vi "OPEN & CONFIG ARMS.vi"(0 "LEFT or RIGHT":string="LEFT", 1 "CLIMBER COAST":T2=enum."Override to Brake", 5 "CLIMBER CAN ID":u8=9, 7 "LOCK PWM channel":T1=enum."PWM 2", 9 "ARM CAN ID":u8=11, 11 "error in (no error)":errorcluster, 12 "Invert climber?":bool, 14 "Invert arm actuator?":bool) -> (15 "error out":errorcluster)   [LabVIEW 2020]
uses:
  <vilib>/Rock Robotics/WPI/ThirdParty/Phoenix-LabVIEW/Motor Controller/Controls/CTRE_Phoenix_MotorControl_TalonFXMotorControllerConfigurables.ctl
  <vilib>/Rock Robotics/WPI/ThirdParty/Phoenix-LabVIEW/Motor Controller/Controls/CTRE_Phoenix_MotorControl_BaseConfigurables.ctl
  <vilib>/Rock Robotics/WPI/ThirdParty/Phoenix-LabVIEW/Motor Controller/Controls/CTRE_Phoenix_MotorControl_VelocityMeasurementPeriod.ctl
  <vilib>/Rock Robotics/WPI/ThirdParty/Phoenix-LabVIEW/Motor Controller/Controls/CTRE_Phoenix_MotorControl_SlotStructure.ctl
  <vilib>/Rock Robotics/WPI/ThirdParty/Phoenix-LabVIEW/Motor Controller/Controls/CTRE_Phoenix_MotorControl_FilterStruct.ctl
  <vilib>/Rock Robotics/WPI/ThirdParty/Phoenix-LabVIEW/Motor Controller/Controls/CTRE_Phoenix_MotorControl_RemoteSourceType.ctl
  <vilib>/Rock Robotics/WPI/ThirdParty/Phoenix-LabVIEW/Controls/CTRE_Phoenix_CustomParamConfiguration.ctl
  <vilib>/Rock Robotics/WPI/ThirdParty/Phoenix-LabVIEW/Motor Controller/Controls/CTRE_Phoenix_MotorControl_FeedbackDevice_TalonFX.ctl
  <vilib>/Rock Robotics/WPI/ThirdParty/Phoenix-LabVIEW/Motor Controller/Controls/CTRE_Phoenix_MotorControl_LimitSwitchNormal.ctl
  <vilib>/Rock Robotics/WPI/ThirdParty/Phoenix-LabVIEW/Motor Controller/Controls/CTRE_Phoenix_MotorControl_LimitSwitchSource_Local.ctl
  <vilib>/Rock Robotics/WPI/ThirdParty/Phoenix-LabVIEW/Motor Controller/Controls/CTRE_Phoenix_MotorControl_SupplyCurrentLimitConfiguration.ctl
  <vilib>/Rock Robotics/WPI/ThirdParty/Phoenix-LabVIEW/Motor Controller/Controls/CTRE_Phoenix_MotorControl_StatorCurrentLimitConfiguration.ctl
  <vilib>/Rock Robotics/WPI/ThirdParty/Phoenix-LabVIEW/Motor Controller/Controls/CTRE_Phoenix_MotorControl_MotorCommutation_TalonFX.ctl
  <vilib>/Rock Robotics/WPI/ThirdParty/Phoenix-LabVIEW/CANCoder/Controls/CTRE_Phoenix_CANcoder_AbsoluteSensorRange.ctl
  <vilib>/Rock Robotics/WPI/ThirdParty/Phoenix-LabVIEW/CANCoder/Controls/CTRE_Phoenix_CANcoder_SensorInitializationStrategy.ctl
  <vilib>/Rock Robotics/WPI/ThirdParty/Phoenix-LabVIEW/Motor Controller/Controls/CTRE_Phoenix_MotorControl_NeutralMode.ctl
  <vilib>/Rock Robotics/SystemInterfaces/DIO/FPGA_DIOPWMChannel.ctl
  <vilib>/Rock Robotics/WPI/SafetyOutput/WPI_SafetyOutputConfigMenu.ctl
  Robot Global Data.vi
  <vilib>/Rock Robotics/Network Tables/NT Write Number.vi
  <vilib>/Rock Robotics/Network Tables/NT Write Boolean.vi
panel:
  in  "FALCON Climbing config":T3={"Base Configurables"={"openLoopRamp"=0.25, "closedLoopRamp"=0.125, "peakOutputForward"=1.0, "peakOutputReverse"=-1.0, "nominalOutputForward"=0.0, "nominalOutputReverse"=0.0, "neutralDeadband"=0.04, "voltageCompSaturation"=0.0, "voltageMeasurementFilter"=32, "velocityMeasurementPeriod"=100, "velocityMeasurementWindow"=64, "forwardSoftLimitThreshold"=441205, "reverseSoftLimitThreshold"=0, "forwardSoftLimitEnable"=TRUE, "reverseSoftLimitEnable"=TRUE, "slot0"={"P"=0.0, "I"=0.0, "D"=0.0, "F"=0.0, "integralZone"=0.0, "allowableClosedLoopError"=0, "maxIntegralAccumulator"=0.0, "closedLoopPeakOutput"=1.0, "closedLoopPeriod"=1}, "slot1"={"P"=0.0, "I"=0.0, "D"=0.0, "F"=0.0, "integralZone"=0.0, "allowableClosedLoopError"=0, "maxIntegralAccumulator"=0.0, "closedLoopPeakOutput"=1.0, "closedLoopPeriod"=1}, "slot2"={"P"=0.0, "I"=0.0, "D"=0.0, "F"=0.0, "integralZone"=0.0, "allowableClosedLoopError"=0, "maxIntegralAccumulator"=0.0, "closedLoopPeakOutput"=1.0, "closedLoopPeriod"=1}, "slot3"={"P"=0.0, "I"=0.0, "D"=0.0, "F"=0.0, "integralZone"=0.0, "allowableClosedLoopError"=0, "maxIntegralAccumulator"=0.0, "closedLoopPeakOutput"=1.0, "closedLoopPeriod"=1}, "auxPIDPolarity"=FALSE, "remoteFilter0"={"remoteSensorDeviceID"=0, "remoteSensorSource"=enum."Off"}, "remoteFilter1"={"remoteSensorDeviceID"=0, "remoteSensorSource"=enum."Off"}, "motionCruiseVelocity"=0, "motionAcceleration"=0, "motionProfileTrajectoryPeriod"=0, "feedbackNotContinuous"=FALSE, "remoteSensorClosedLoopDisableNeutralOnLOS"=FALSE, "clearPositionOnLimitF"=FALSE, "clearPositionOnLimitR"=FALSE, "clearPositionOnQuadIdx"=FALSE, "limitSwitchDisableNeutralOnLOS"=FALSE, "softLimitDisableNeutralOnLOS"=FALSE, "pulseWidthPeriod_EdgesPerRot"=1, "pulseWidthPeriod_FilterWindowSz"=1, "customParam"={"customParam0"=0, "customParam1"=0}, "trajectoryInterpolationEnable"=TRUE}, "primaryPID"={"selectedFeedbackCoefficient"=1.0, "selectedFeedbackSensor"=1}, "auxiliaryPID"={"selectedFeedbackCoefficient"=1.0, "selectedFeedbackSensor"=1}, "forwardLimitSwitchNormal"=enum."Normally Open", "reverseLimitSwitchNormal"=enum."Normally Open", "forwardLimitSwitchDeviceID"=0, "reverseLimitSwitchDeviceID"=0, "forwardLimitSwitchSource"=enum."Feedback Connector", "reverseLimitSwitchSource"=enum."Feedback Connector", "sum0Term"=1, "sum1Term"=1, "diff0Term"=1, "diff1Term"=1, "Supply Current Limit Configuration"={"Enable?"=FALSE, "Current Limit"=0.0, "Threshold Current"=0.0, "Threshold Time"=0.0}, "Stator Current Limit Configuration"={"Enable?"=FALSE, "Current Limit"=0.0, "Threshold Current"=0.0, "Threshold Time"=0.0}, "Motor Commutation"=enum."Trapezoidal", "Absolute Sensor Range"=enum."Unsigned [0 to 360)", "Integrated Sensor Offset (Degrees)"=0.0, "Sensor Initialization Strategy"=enum."Boot To Zero"} {"diff1Term" items=["Integrated Sensor"=1, "Sensor Sum (S0 + S1)"=9, "Sensor Difference (D0 - D1)"=10, "Remote Source 0"=11, "Remote Source 1"=12, "None"=14, "Software Emulated"=15]; "diff0Term" items=["Integrated Sensor"=1, "Sensor Sum (S0 + S1)"=9, "Sensor Difference (D0 - D1)"=10, "Remote Source 0"=11, "Remote Source 1"=12, "None"=14, "Software Emulated"=15]; "sum1Term" items=["Integrated Sensor"=1, "Sensor Sum (S0 + S1)"=9, "Sensor Difference (D0 - D1)"=10, "Remote Source 0"=11, "Remote Source 1"=12, "None"=14, "Software Emulated"=15]; "sum0Term" items=["Integrated Sensor"=1, "Sensor Sum (S0 + S1)"=9, "Sensor Difference (D0 - D1)"=10, "Remote Source 0"=11, "Remote Source 1"=12, "None"=14, "Software Emulated"=15]; "auxiliaryPID"."selectedFeedbackSensor" items=["Integrated Sensor"=1, "Sensor Sum (S0 + S1)"=9, "Sensor Difference (D0 - D1)"=10, "Remote Source 0"=11, "Remote Source 1"=12, "None"=14, "Software Emulated"=15]; "primaryPID"."selectedFeedbackSensor" items=["Integrated Sensor"=1, "Sensor Sum (S0 + S1)"=9, "Sensor Difference (D0 - D1)"=10, "Remote Source 0"=11, "Remote Source 1"=12, "None"=14, "Software Emulated"=15]; "Base Configurables"."velocityMeasurementPeriod" items=["Period_1ms"=1, "Period_2ms"=2, "Period_5ms"=5, "Period_10ms"=10, "Period_20ms"=20, "Period_25ms"=25, "Period_50ms"=50, "Period_100ms"=100]}
  # "Climbing soft limit calc:\n23.5\" max travel\n1.25\" diameter sprocket\n36:1 planetary gearbox\n2048 encoder tics/rev for a Falcon 500\n\n23.5 in * rev/(pi*1.25\") * 36 motor rev/rev * 2048 tics/motor rev = 441205 tics"
  # "Sum and Diff terms are ways to select more than one sensor as a feedback device. \n Sum 0 is the first feedback device to be used for the Sum term.\n Sum 1 is the feedback device to be added to Sum 0 for the Sum term.\n Diff 0 and Diff 1 work in a similar manner."
  # "These are only applicable\nif using a remote limit switch.\n\nLocal limit switches/no limit\nswitches do not use this."
  # "Current is below Current Limit AND\n\n(Requested output is weaker** than applied motor\noutput OR is in the opposite direction).\n/\nMotor output is set to requested output."
  # "Current is above Threshold Current for Threshold Time\n/\nReduce motor output (towards neutral)."
  # "Current is below Current Limit.\n/\nRamp motor output towards requested output."
  # "Current is above Current Limit.\n/\nReduce motor output (towards neutral)."
  # "*If the configured Peak Threshold is less than the Continuous Threshold, the applied Peak Threshold is set equal to the Configured Continuous Threshold in firmware.\n** Both requested output and applied motor output are in the same direction, and requested output is closer to neutral."
  # "False: Primary Output = PID[0] + PID[1]  ---  Auxiliary Output = PID[0] - PID[1]\nTrue:  Primary Output = PID[0] - PID[1] --- Auxiliary Output = PID[0] + PID[1]"
  # "Enable the motion profile executor to perform linear interpolation between profile points.  Defaults to True."
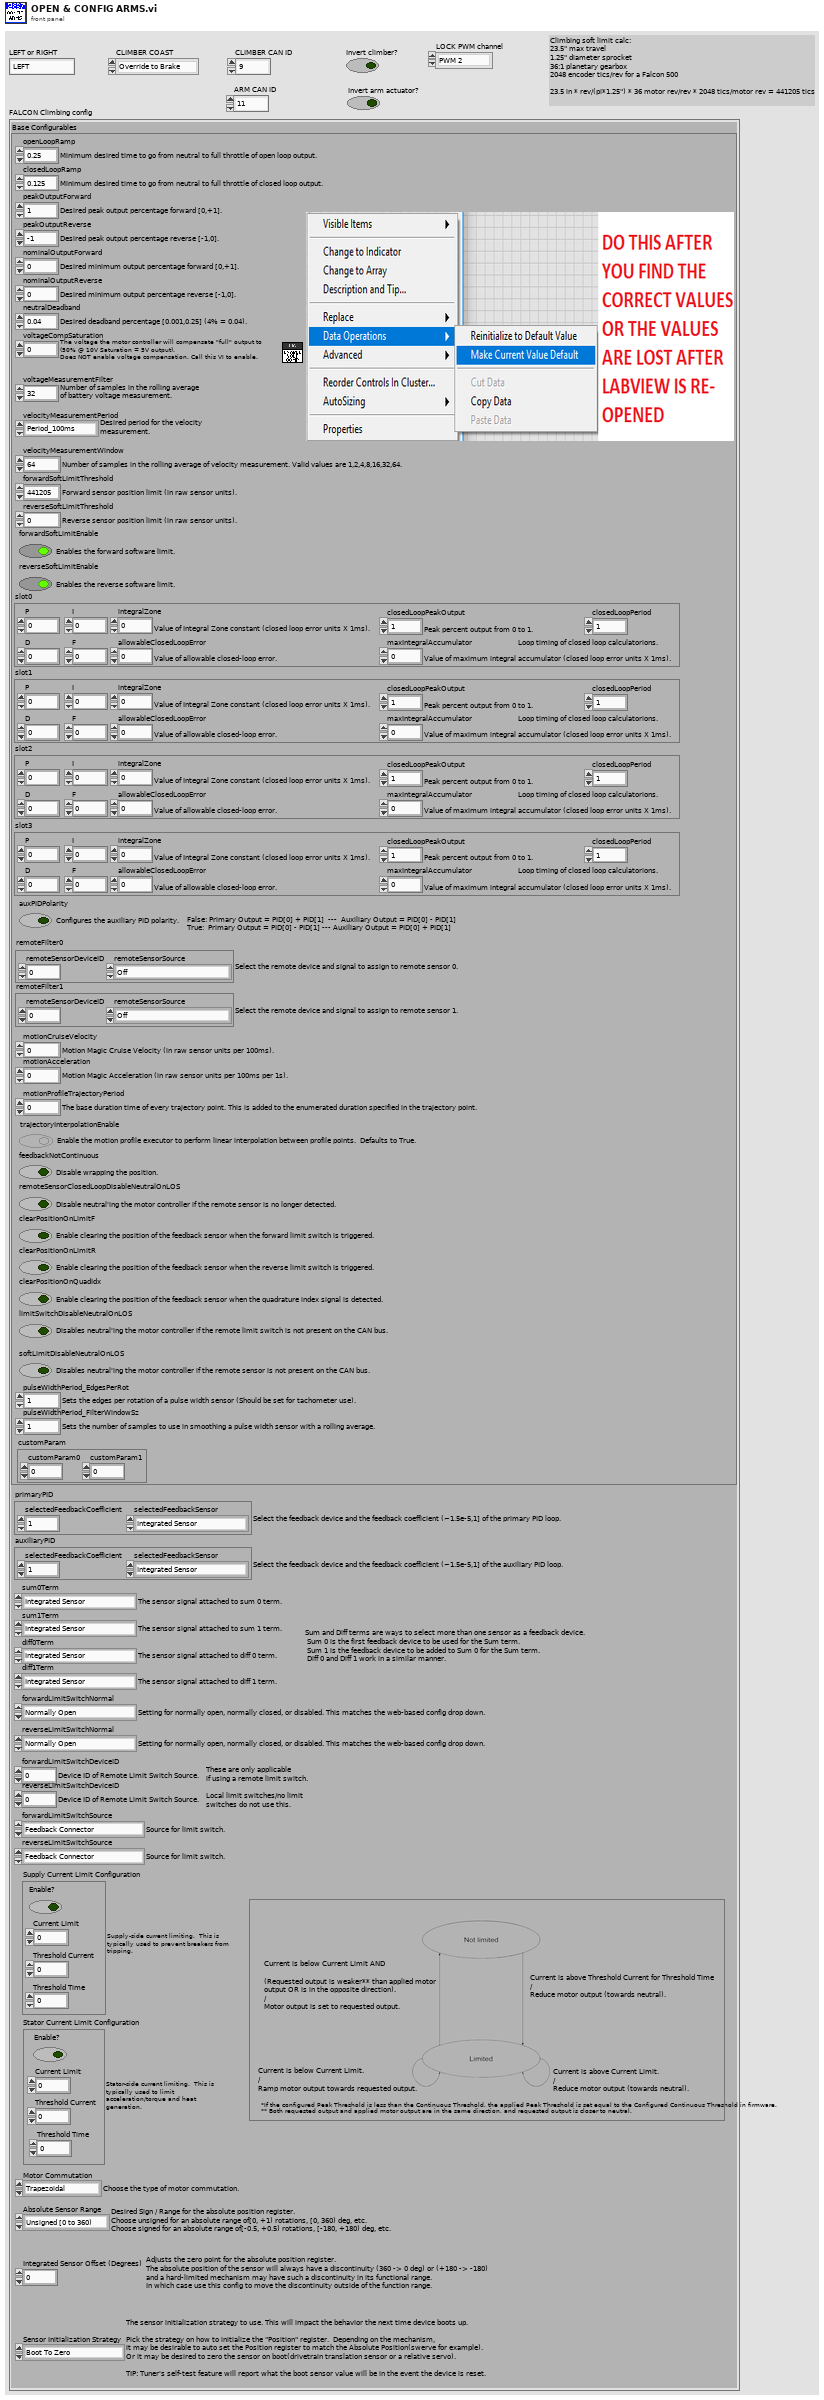
[diagram p1: front panel]
types:
  T1 = typedef "FPGA_DIOPWMChannel.ctl" = enum8{"PWM 0", "PWM 1", "PWM 2", "PWM 3", "PWM 4", "PWM 5", "PWM 6", "PWM 7", "PWM 8", "PWM 9", "PWM MXP 0", "PWM MXP 1", "PWM MXP 2", "PWM MXP 3", "PWM MXP 4", "PWM MXP 5", "PWM MXP 6", "PWM MXP 7", "PWM MXP 8", "PWM MXP 9", "Invalid"}
  T2 = typedef "CTRE_Phoenix_MotorControl_NeutralMode.ctl" = enum8{"EEPROMSetting", "Override to Coast", "Override to Brake"}
  T3 = typedef "CTRE_Phoenix_MotorControl_TalonFXMotorControllerConfigurables.ctl" = cluster{"Base Configurables":T4, "primaryPID":cluster{"selectedFeedbackCoefficient":dbl, "selectedFeedbackSensor":T10}, "auxiliaryPID":cluster{"selectedFeedbackCoefficient":dbl, "selectedFeedbackSensor":T10}, "forwardLimitSwitchNormal":T11, "reverseLimitSwitchNormal":T11, "forwardLimitSwitchDeviceID":i32, "reverseLimitSwitchDeviceID":i32, "forwardLimitSwitchSource":T12, "reverseLimitSwitchSource":T12, "sum0Term":T10, "sum1Term":T10, "diff0Term":T10, "diff1Term":T10, "Supply Current Limit Configuration":T13, "Stator Current Limit Configuration":T14, "Motor Commutation":T15, "Absolute Sensor Range":T16, "Integrated Sensor Offset (Degrees)":dbl, "Sensor Initialization Strategy":T17}
  T4 = typedef "CTRE_Phoenix_MotorControl_BaseConfigurables.ctl" = cluster{"openLoopRamp":dbl, "closedLoopRamp":dbl, "peakOutputForward":dbl, "peakOutputReverse":dbl, "nominalOutputForward":dbl, "nominalOutputReverse":dbl, "neutralDeadband":dbl, "voltageCompSaturation":dbl, "voltageMeasurementFilter":i32, "velocityMeasurementPeriod":T5, "velocityMeasurementWindow":i32, "forwardSoftLimitThreshold":i32, "reverseSoftLimitThreshold":i32, "forwardSoftLimitEnable":bool, "reverseSoftLimitEnable":bool, "slot0":T6, "slot1":T6, "slot2":T6, "slot3":T6, "auxPIDPolarity":bool, "remoteFilter0":T7, "remoteFilter1":T7, "motionCruiseVelocity":i32, "motionAcceleration":i32, "motionProfileTrajectoryPeriod":i32, "feedbackNotContinuous":bool, "remoteSensorClosedLoopDisableNeutralOnLOS":bool, "clearPositionOnLimitF":bool, "clearPositionOnLimitR":bool, "clearPositionOnQuadIdx":bool, "limitSwitchDisableNeutralOnLOS":bool, "softLimitDisableNeutralOnLOS":bool, "pulseWidthPeriod_EdgesPerRot":i32, "pulseWidthPeriod_FilterWindowSz":i32, "customParam":T9, "trajectoryInterpolationEnable":bool}
  T5 = typedef "CTRE_Phoenix_MotorControl_VelocityMeasurementPeriod.ctl" = u16
  T6 = typedef "CTRE_Phoenix_MotorControl_SlotStructure.ctl" = cluster{"P":dbl, "I":dbl, "D":dbl, "F":dbl, "integralZone":dbl, "allowableClosedLoopError":i32, "maxIntegralAccumulator":dbl, "closedLoopPeakOutput":dbl, "closedLoopPeriod":i32}
  T7 = typedef "CTRE_Phoenix_MotorControl_FilterStruct.ctl" = cluster{"remoteSensorDeviceID":u8, "remoteSensorSource":T8}
  T8 = typedef "CTRE_Phoenix_MotorControl_RemoteSourceType.ctl" = enum16{"Off", "Talon SRX Selected Sensor", "Pigeon IMU Yaw", "Pigeon IMU Pitch", "Pigeon IMU Roll", "CANifier Quadrature", "CANifier PWM Input 0", "CANifier PWM Input 1", "CANifier PWM Input 2", "CANifier PWM Input 3", "Gadgeteer Pigeon Yaw", "Gadgeteer Pigeon Pitch", "Gadgeteer Pigeon Roll", "CANCoder"}
  T9 = typedef "CTRE_Phoenix_CustomParamConfiguration.ctl" = cluster{"customParam0":i32, "customParam1":i32}
  T10 = typedef "CTRE_Phoenix_MotorControl_FeedbackDevice_TalonFX.ctl" = i8
  T11 = typedef "CTRE_Phoenix_MotorControl_LimitSwitchNormal.ctl" = enum16{"Normally Open", "Normally Closed", "Disabled"}
  T12 = typedef "CTRE_Phoenix_MotorControl_LimitSwitchSource_Local.ctl" = enum16{"Feedback Connector", "Remote Talon SRX", "Remote CANifier", "Deactivated"}
  T13 = typedef "CTRE_Phoenix_MotorControl_SupplyCurrentLimitConfiguration.ctl" = cluster{"Enable?":bool, "Current Limit":dbl, "Threshold Current":dbl, "Threshold Time":dbl}
  T14 = typedef "CTRE_Phoenix_MotorControl_StatorCurrentLimitConfiguration.ctl" = cluster{"Enable?":bool, "Current Limit":dbl, "Threshold Current":dbl, "Threshold Time":dbl}
  T15 = typedef "CTRE_Phoenix_MotorControl_MotorCommutation_TalonFX.ctl" = enum16{"Trapezoidal"}
  T16 = typedef "CTRE_Phoenix_CANcoder_AbsoluteSensorRange.ctl" = enum16{"Unsigned [0 to 360)", "Signed [-180 to +180)"}
  T17 = typedef "CTRE_Phoenix_CANcoder_SensorInitializationStrategy.ctl" = enum16{"Boot To Zero", "Boot To Absolute Position"}
  T18 = typedef "WPI_SafetyOutputConfigMenu.ctl" = enum16{"Enable", "Disable"}
  T19 = typedef "WPI_MotorControlDeviceRef.ctl" = cluster{"DeviceStatus":errorcluster, "Type":T20, "PWM":cluster{"PWM Channel":T1, "DeadBand":T21}, "CAN":cluster{"Device Number":u8, "SetOutput VI Ref":variant, "GetOutput VI Ref":variant, "Enable VI Ref":variant, "Disable VI Ref":variant, "Data":variant}, "Invert":bool, "DIO PWM":cluster{"PWM \"Enable\" Channel":T1, "DIOChannel":T22, "PWM Rate":dbl}}
  T20 = typedef "WPI_MotorControlType.ctl" = enum16{"PWM", "CAN", "DIO PWM"}
  T21 = typedef "WPI_PWMDeadband.ctl" = cluster{"Name":string, "maxPositivePwm":i32, "minPositivePwm":i32, "centerPwm":i32, "maxNegativePwm":i32, "minNegativePwm":i32, "angularRange":u16}
  T22 = typedef "FPGA_DIOChannel.ctl" = enum8{"DIO 0", "DIO 1", "DIO 2", "DIO 3", "DIO 4", "DIO 5", "DIO 6", "DIO 7", "DIO 8", "DIO 9", "DIO MXP 0", "DIO MXP 1", "DIO MXP 2", "DIO MXP 3", "DIO MXP 4", "DIO MXP 5", "DIO MXP 6", "DIO MXP 7", "DIO MXP 8", "DIO MXP 9", "DIO MXP 10", "DIO MXP 11", "DIO MXP 12", "DIO MXP 13", "DIO MXP 14", "DIO MXP 15", "SPI Port CS1", "SPI Port CS2", "SPI Port CS3", "SPI Port MISO", "SPI Port MOSI", "Invalid"}
  T23 = cluster{"MIN":dbl, "MAX":dbl, "convert climber inches to tics":dbl}
  T24 = cluster{"RANGE":u16, "UNLOCKED angle":i32, "LOCKED angle":i32}
  T25 = typedef "WPI_ServoDeviceRef.ctl" = cluster{"DeviceStatus":errorcluster, "PWM Channel":T1, "DeadBand":T21}
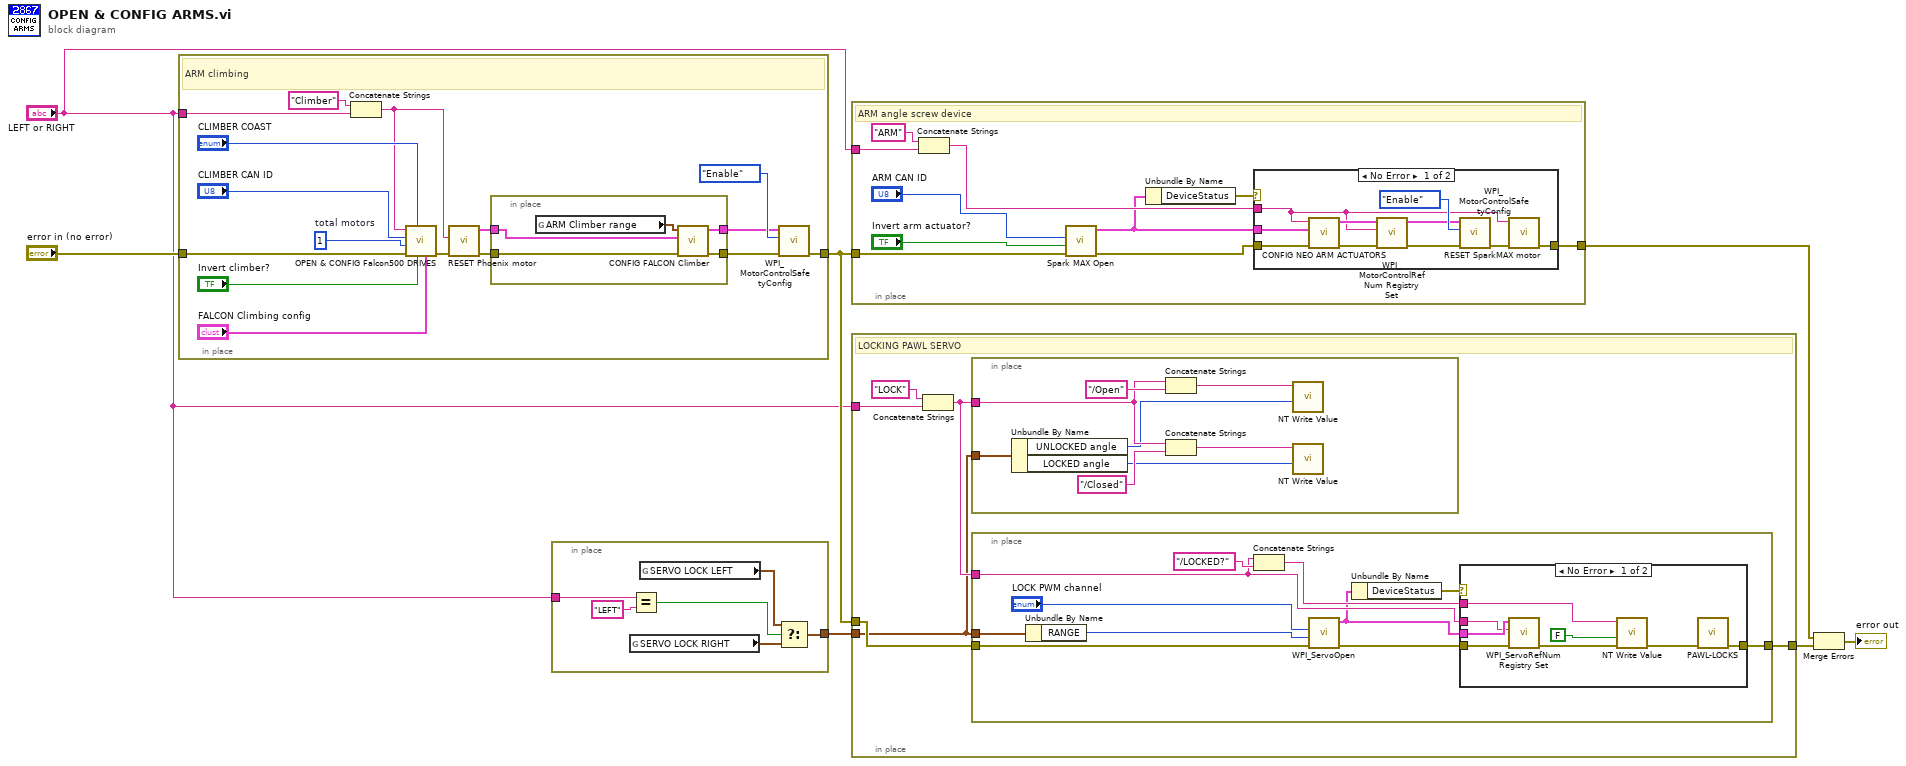
[diagram p0: block diagram]
diagram:
  n1 = in-place {
    in-place-border: "error in (no error)" -> [w14]
    in-place-border: "LEFT or RIGHT" -> [w23]
    in-place-border: [w21] -> w5
    w18 = 1  # total motors
    # "ARM climbing"
    n2 = Concatenate Strings("Climber" ("refnum name"), w23) -> (w12:string)
    n3 = call "OPEN & CONFIG Falcon500 DRIVES.vi"("Talon FX Configurables"="FALCON Climbing config", "INVERT motors?"="Invert climber?", "Motor Control Neutral Mode"="CLIMBER COAST", "error in"=w14, "total motors"=w18, "CAN ID for MASTER DRIVE"="CLIMBER CAN ID", "MASTER DRIVE REF name"=w12) -> ("error out"=w13:errorcluster)  [unwired: 2 in, 2 out]
    n4 = call "RESET Phoenix motor.vi"("error in (no error)"=w13, "Phoenix motor refname"=w12) -> ("error out"=w9:errorcluster, "PhoenixMotorControlDevRef"=w11:T19)  [unwired: 6 in, 2 out]
    n5 = in-place {
      in-place-border: w11 -> [w28]
      in-place-border: [w26] -> w10
      in-place-border: w9 -> [w25]
      in-place-border: [w24] -> w8
      n6 = global read "Robot Global Data.vi" "ARM Climber range"() -> (w27:T23)
      n7 = call "CONFIG FALCON Climber.vi"("error in (no error)"=w25, "PhoenixMotorControlDevRef in"=w28, "ARM Climber range"=w27) -> ("error out"=w24:errorcluster, "PhoenixMotorControlDevRef out"=w26:T19)  [unwired: 7 in]
    }
    n8 = call <vilib>:"WPI_MotorControlSafetyConfig.vi"("error in (no error)"=w8, "mode"=WPI_SafetyOutputConfigMenu."Enable", "MotorControlDevRef"=w10) -> ("error out"=w21:errorcluster)  [unwired: 7 in, 1 out]
  }
  n9 = in-place {
    in-place-border: "LEFT or RIGHT" -> [w33]
    in-place-border: [w29] -> w1
    n10 = global read "Robot Global Data.vi" "SERVO LOCK RIGHT"() -> (w30:T24)
    n11 = Equal?(x=w33, y="LEFT") -> (x = y?=w34:bool)
    n12 = global read "Robot Global Data.vi" "SERVO LOCK LEFT"() -> (w31:T24)
    n13 = Select(t=w31, s=w34, f=w30) -> (s? t:f=w29:T24)
  }
  n14 = in-place "In Place Element Structure" {
    in-place-border: "LEFT or RIGHT" -> [w44]
    in-place-border: [w38] -> w6
    in-place-border: w5 -> [w42]
    # "ARM angle screw device"
    n15 = Concatenate Strings("ARM" ("refnum name"), w44) -> (w37:string)
    n16 = call <vilib>:"Spark MAX Open.vi"("error in (no error)"=w42, "Invert"="Invert arm actuator?", "Device Number"="ARM CAN ID") -> ("error out"=w39:errorcluster, "MotorControlDeviceRef"=w35:T19)  [unwired: 7 in]
    n17 = Unbundle By Name(w35) -> ("DeviceStatus"=w36:errorcluster)
    n18 = case shown="No Error" w36 {
      tunnel: w39 -> [w51 _]
      tunnel: w35 -> [w50 _]
      tunnel: [w46 _] -> w38
      tunnel: w37 -> [w45 _]
      frame No Error {
        n19 = call "CONFIG NEO ARM ACTUATORS.vi"("error in (no error)"=w51, "MotorControlDevRef"=w50, "RefName"=w45) -> ("error out"=w52:errorcluster, "MotorControlDeviceRef out"=w49:T19)  [unwired: 7 in]
        n20 = call <vilib>:"WPI_MotorControlRefNum Registry Set.vi"("error in (no error)"=w52, "refnum name"=w45, "MotorControlDevRef"=w49) -> ("error out"=w48:errorcluster, "MotorControlDevRef"=w53:T19)  [unwired: 7 in]
        n21 = call <vilib>:"WPI_MotorControlSafetyConfig.vi"("error in (no error)"=w48, "mode"=WPI_SafetyOutputConfigMenu."Enable", "MotorControlDevRef"=w53) -> ("error out"=w47:errorcluster)  [unwired: 7 in, 1 out]
        n22 = call "RESET SparkMAX motor.vi"("error in (no error)"=w47, "SparkMAX motor refname"=w45) -> ("error out"=w46:errorcluster)  [unwired: 6 in, 3 out]
      }
      frame Error {
      }
    }
  }
  n23 = in-place {
    in-place-border: "LEFT or RIGHT" -> [w59]
    in-place-border: [w56] -> w3
    in-place-border: w5 -> [w58]
    in-place-border: w1 -> [w55]
    # "LOCKING PAWL SERVO"
    n24 = Concatenate Strings("LOCK" ("refnum name"), w59) -> (w57:string)
    n25 = in-place {
      in-place-border: w57 -> [w64]
      in-place-border: w55 -> [w61]
      n26 = Unbundle By Name(w61) -> ("UNLOCKED angle"=w62:i32, "LOCKED angle"=w63:i32)
      n27 = Concatenate Strings(w64, "/Open" ("string")) -> (w68:string)
      n28 = Concatenate Strings(w64, "/Closed" ("string")) -> (w66:string)
      n29 = call-poly <vilib>:"NT Write Value.vi"("Numeric"=w62, "Name"=w68) -> ()  [unwired: 9 in, 1 out]
      n30 = call-poly <vilib>:"NT Write Value.vi"("Numeric"=w63, "Name"=w66) -> ()  [unwired: 9 in, 1 out]
    }
    n31 = in-place {
      in-place-border: w58 -> [w77]
      in-place-border: w57 -> [w74]
      in-place-border: [w73] -> w56
      in-place-border: w55 -> [w71]
      n32 = Unbundle By Name(w71) -> ("RANGE"=w72:u16)
      n33 = Concatenate Strings(w74, "/LOCKED?" ("string")) -> (w76:string)
      n34 = call <vilib>:"WPI_ServoOpen.vi"("error in (no error)"=w77, "Angular Range"=w72, "PWM Channel"="LOCK PWM channel") -> ("error out"=w78:errorcluster, "ServoDeviceRef"=w69:T25)  [unwired: 7 in]
      n35 = Unbundle By Name(w69) -> ("DeviceStatus"=w70:errorcluster)
      n36 = case shown="No Error" w70 {
        tunnel: w78 -> [w87 _]
        tunnel: w69 -> [w86 _]
        tunnel: w76 -> [w84 _]
        tunnel: w74 -> [w83 _]
        tunnel: [w82 _] -> w73
        frame No Error {
          n37 = call <vilib>:"WPI_ServoRefNum Registry Set.vi"("error in (no error)"=w87, "refnum name"=w83, "ServoDeviceRef"=w86) -> ("error out"=w81:errorcluster)  [unwired: 7 in, 1 out]
          n38 = call-poly <vilib>:"NT Write Value.vi"("error in"=w81, "Boolean"=FALSE, "Name"=w84) -> ("error out"=w80:errorcluster)  [unwired: 8 in]
          n39 = call "PAWL-LOCKS.vi"("error in"=w80) -> ("error out"=w82:errorcluster)  [unwired: 8 in, 2 out]
        }
        frame Error {
        }
      }
    }
  }
  n40 = Merge Errors(w6, w3) -> (→"error out":errorcluster)
